vi "Main.vi"(11 "Module Admin":refnum<class "Delacor_lib_QMH_Cloneable Module Admin.lvclass">) -> ()   [LabVIEW 2020, in "reporting-device.lvlib"]
doc: "This template is based off of the Queued Message Handler design pattern and the Queued Message Handler project template that ships with LabVIEW.\n\nThe main difference is that the queue is private to this module and communication between modules is performed via Broadcast and Request events.\n\nRequest events are wrapped in public API methods and are handled in the Event Handling Loop (EHL) of this VI. Any module can register for Broadcast events sent by this module. The EHL generates messages based on user interface actions.\n\nThe Message Handling Loop (MHL) processes messages generated by the EHL, or by other messages. The messages are string values, so new messages can be added easily to the Message Cases case structure in the MHL. Each message cluster can also provide an optional value for Message Data, which is a variant that can be converted to whatever message-specific data is required.\n_____\nBased on DQMH Project Template 7.0.1.1316."
uses:
  reporting-device.lvlib
  <vilib>/Delacor/Delacor QMH/Libraries/Cloneable Module Admin_class/Delacor_lib_QMH_Cloneable Module Admin.lvclass
  C:/Program Files (x86)/National Instruments/LabVIEW 2020/vi.lib/Delacor/Delacor QMH/Libraries/Module Admin_class/Delacor_lib_QMH_Module Admin.lvclass
  <vilib>/Delacor/Delacor QMH/Libraries/Cloneable Module Admin_class/Delacor_lib_QMH_Cloneable Module Admin.lvclass/Delacor_lib_QMH_Cloneable Module Admin.ctl
  <vilib>/Wovalab/Utilities/Helper Loop Periodic Timing/Helper Loop Periodic Timing.lvclass/Helper Loop Periodic Timing.ctl
  <userlib>/Zaphiro/GTools/Redis/Sources/Redis/Redis.lvclass/Redis.ctl
  Stop Argument--cluster.ctl
  <vilib>/Delacor/Delacor QMH/Libraries/Message Queue_class/Delacor_lib_QMH_Message Queue.lvclass/Delacor_lib_QMH_Message Queue.ctl
  <vilib>/Delacor/Delacor QMH/Libraries/Module Admin_class/Delacor_lib_QMH_Module Admin.lvclass/Delacor_lib_QMH_Module Admin.ctl
  connect Argument--cluster.ctl
  connect (Reply Payload)--cluster.ctl
  start-publishing Argument--cluster.ctl
  start-publishing (Reply Payload)--cluster.ctl
  set-reporting-device Argument--cluster.ctl
  set-reporting-device (Reply Payload)--cluster.ctl
  <vilib>/Utility/miscctls.llb/LVPointTypeDef.ctl
  <vilib>/Delacor/Delacor QMH/Libraries/Cloneable Module Admin_class/Delacor_lib_QMH_Get Module ID.vi
  <vilib>/Delacor/Delacor QMH/Libraries/Message Queue_class/Delacor_lib_QMH_Enqueue Message (Single).vi
  <vilib>/Delacor/Delacor QMH/Libraries/Module Admin_class/Delacor_lib_QMH_Get External Launch.vi
  <userlib>/Zaphiro/GTools/Time/public/convert lv time to unix-scalar__ZGTools.vi
  <vilib>/Wovalab/Utilities/Helper Loop Periodic Timing/U32 Max Value--constant.vi
  <userlib>/Zaphiro/GTools/Redis/Sources/Redis/Hashes/HSET.vi
  <userlib>/Zaphiro/GTools/Redis/Sources/Redis/Keys/EXPIRE.vi
  <vilib>/Wovalab/Utilities/Helper Loop Periodic Timing/Update Last Execution Time.vi
  <vilib>/Wovalab/Utilities/Helper Loop Periodic Timing/Stop Helper Loop.vi
  <vilib>/Wovalab/Utilities/Helper Loop Periodic Timing/Stop Helper Loop Internal.vi
  <userlib>/Zaphiro/GTools/Redis/Sources/Redis/Connection/Send-command.vi
  <userlib>/Zaphiro/GTools/Redis/Sources/Redis/Connection/PING.vi
  <userlib>/Zaphiro/GTools/Redis/Sources/Redis/Connection/QUIT.vi
  <vilib>/Wovalab/Utilities/Helper Loop Periodic Timing/Loops Events AE.vi
  <vilib>/Wovalab/Utilities/Helper Loop Periodic Timing/Notify Monitoring Window.vi
  <vilib>/Wovalab/Utilities/Helper Loop Periodic Timing/Monitoring--global.vi
  <userlib>/Zaphiro/GTools/Redis/Sources/Redis/subVIs/LL_collect-response.vi
  <vilib>/Wovalab/Utilities/Helper Loop Periodic Timing/Helper Loop Periodic Timing.lvclass
  <userlib>/Zaphiro/GTools/Redis/Sources/Redis/Redis.lvclass
  <vilib>/Delacor/Delacor QMH/Libraries/Message Queue_class/Delacor_lib_QMH_Message Queue.lvclass
  <userlib>/Zaphiro/GTools/Time/time__ZGTools.lvlib
  <userlib>/Zaphiro/GTools/Time/public/convert unix time to lv-scalar__ZGTools.vi
panel:
  out "values":dbl[](array[numeric])
  out "timestamp":timestamp format="%^<%x %.3X>T utc"
  out "latest-ts":u64
  out "info":T1
  out "status":string
  out "connected":bool
  out "error out":errorcluster
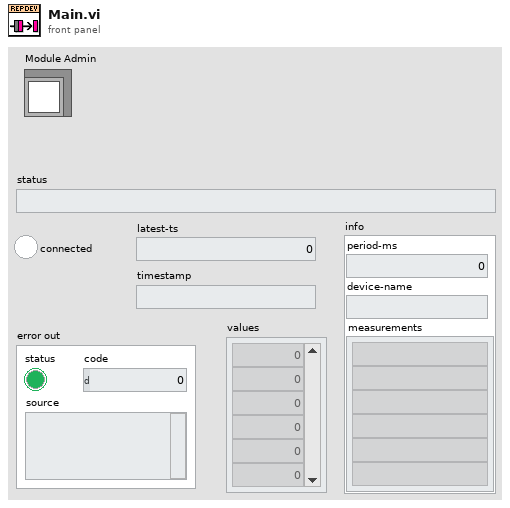
[diagram p1: front panel]
types:
  T1 = cluster{"period-ms":i32, "device-name":string, "measurements":string[]}
  T2 = typedef "reporting-device.lvlib/Request Events--cluster.ctl" = cluster{"Stop Module":refnum<user-event>, "Show Panel":refnum<user-event>, "Hide Panel":refnum<user-event>, "Show Diagram":refnum<user-event>, "Get Module Execution Status":refnum<user-event>, "connect":refnum<user-event>, "start-publishing":refnum<user-event>, "set-reporting-device":refnum<user-event>}
  T3 = typedef "reporting-device.lvlib/Module Data--cluster.ctl" = cluster{"clone-id":i32, "status":string, "dvr":cluster{"redis":refnum<data-value>}}
  T4 = enum32{"invalid lock state", "Not Locked", "Locked (No Password)", "Password-protected"}
  T5 = typedef "reporting-device.lvlib/Stop Argument--cluster.ctl" = cluster{"Module ID":i32, "Origin":string, "Exit via Stop Module Req?":bool, "Wait for Module to stop?":bool}
  T6 = typedef "reporting-device.lvlib/connect Argument--cluster.ctl" = cluster{"Module ID":i32, "flush":bool, "connection":cluster{"ip":string, "port":u16, "timeout":i32}, "Wait Notifier":refnum<notifier>, "wait for reply":bool}
  T7 = typedef "reporting-device.lvlib/start-publishing Argument--cluster.ctl" = cluster{"Module ID":i32, "Wait Notifier":refnum<notifier>, "wait for reply":bool}
  T8 = typedef "reporting-device.lvlib/set-reporting-device Argument--cluster.ctl" = cluster{"Module ID":i32, "measurement-list":string[], "period-ms":i32, "device-name":string, "Wait Notifier":refnum<notifier>, "wait for reply":bool}
  T9 = typedef "LVPointTypeDef.ctl" = cluster{"Horizontal":i16, "Vertical":i16}
  T10 = enum32{"Invalid", "Standard", "Closed", "Hidden", "Minimized", "Maximized"}
  T11 = typedef "reporting-device.lvlib/connect (Reply Payload)--cluster.ctl" = cluster{"Module ID":i32, "status":cluster{"reply-to-ping":bool, "pong":bool}, "error":errorcluster}
  T12 = typedef "reporting-device.lvlib/start-publishing (Reply Payload)--cluster.ctl" = cluster{"Module ID":i32, "ack":bool, "ts":u64, "error":errorcluster}
  T13 = typedef "reporting-device.lvlib/set-reporting-device (Reply Payload)--cluster.ctl" = cluster{"Module ID":i32, "ack":bool, "error":errorcluster}
  T14 = cluster{"output cluster":refnum<class "Redis.lvclass">}
  T15 = cluster{"period-ms":i32, "device-name":string, "measurement-list":string[]}
  T16 = cluster{u64, "device-name":string, "measurement-list":string[]}
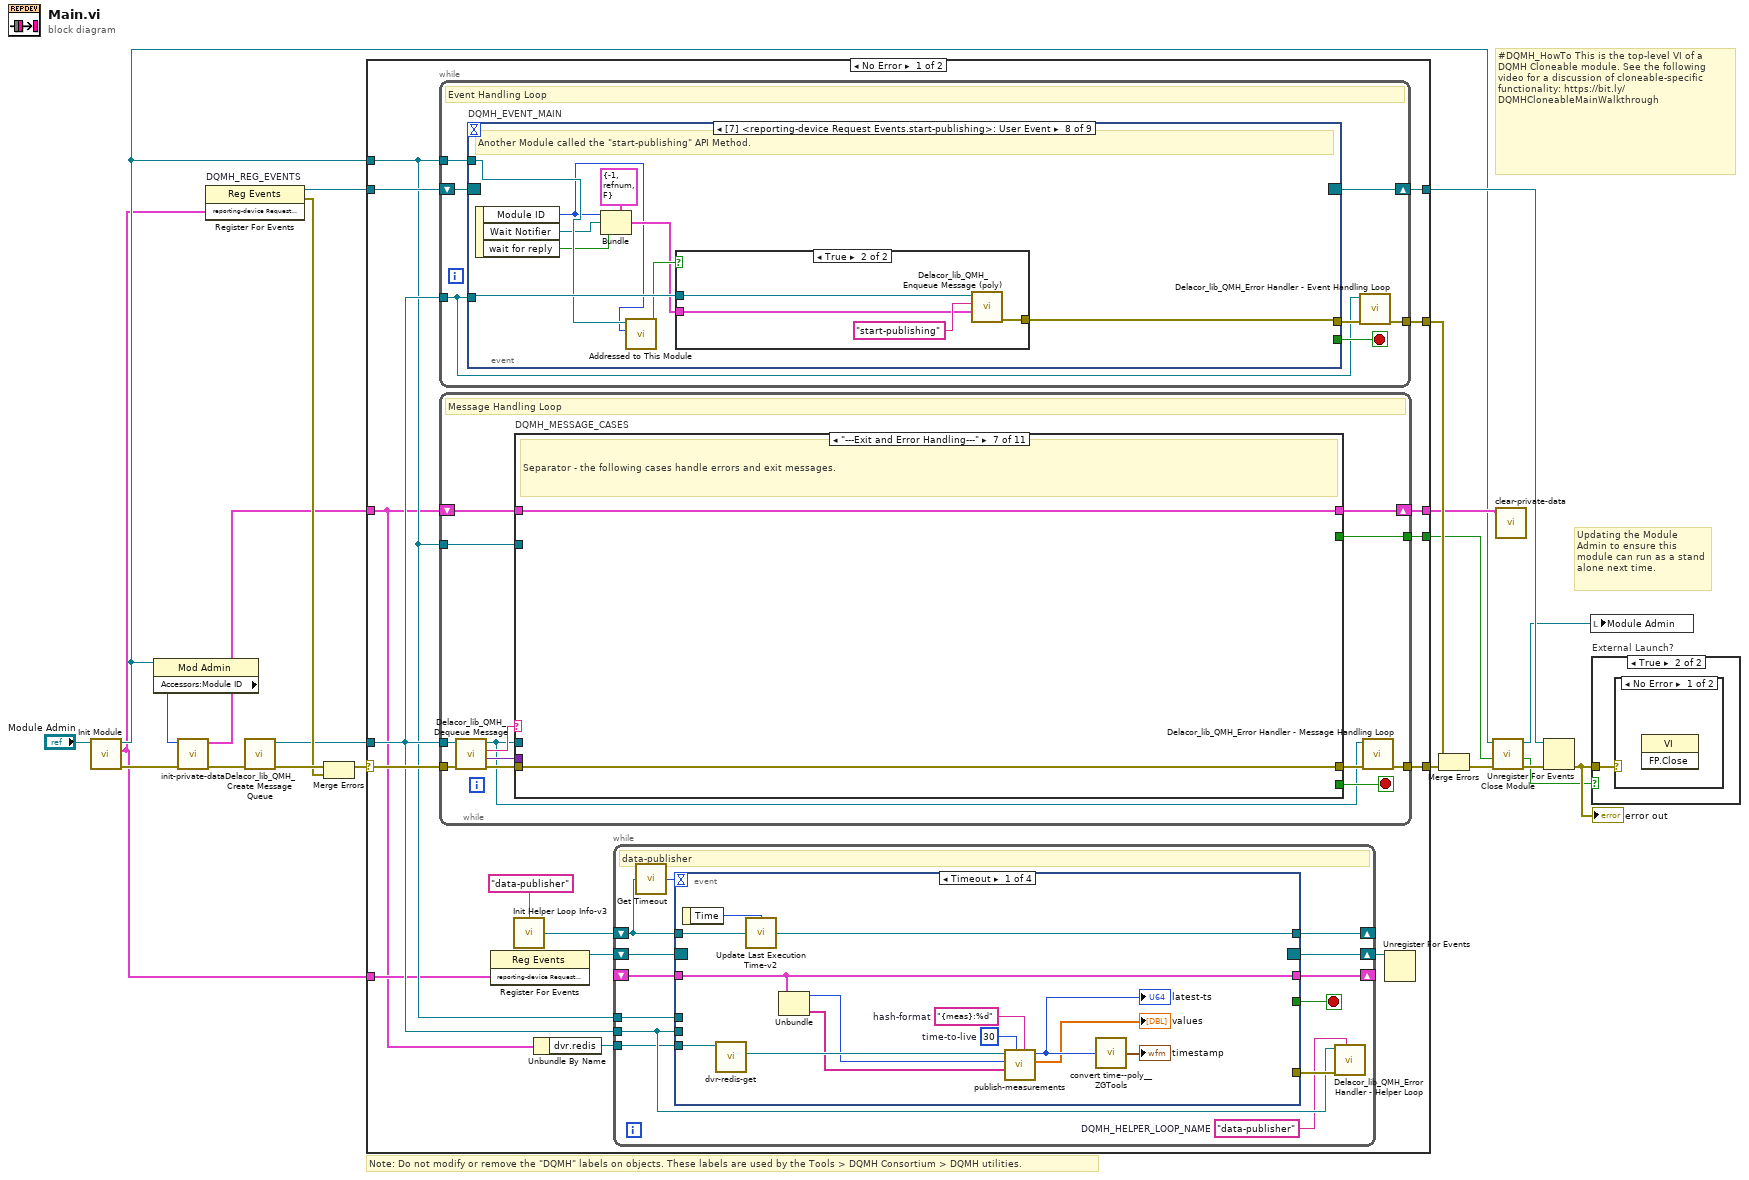
[diagram p0: block diagram]
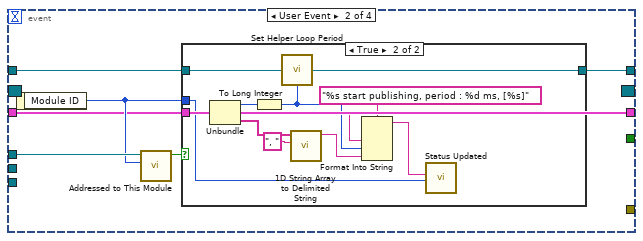
[diagram p2: hidden frame]
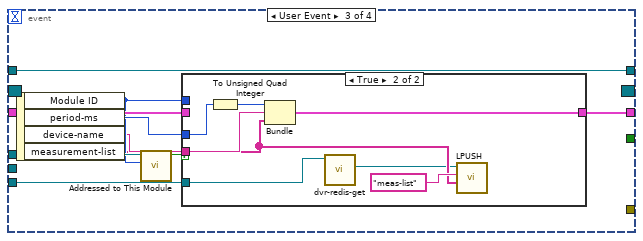
[diagram p4: hidden frame]
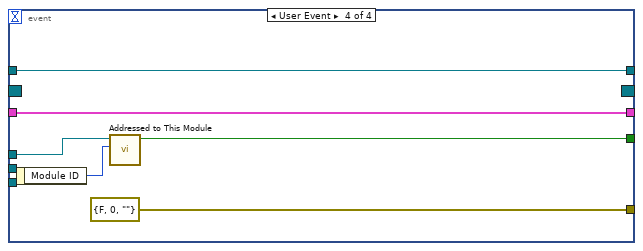
[diagram p6: hidden frame]
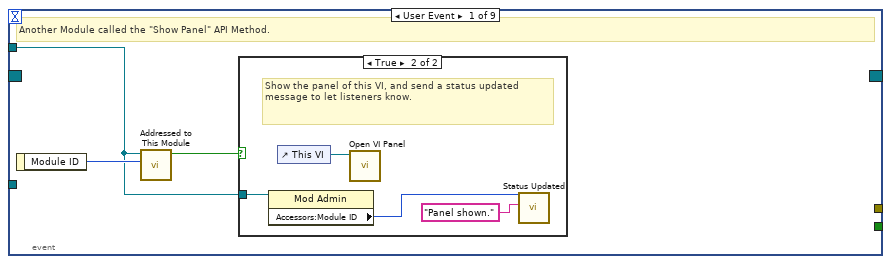
[diagram p7: hidden frame]
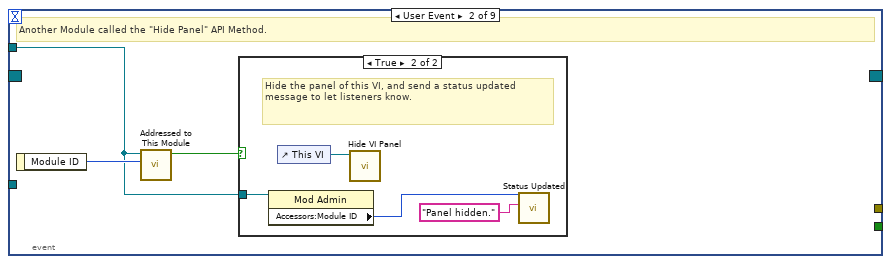
[diagram p9: hidden frame]
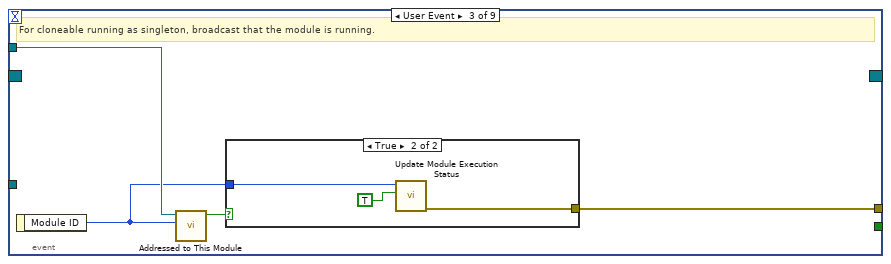
[diagram p11: hidden frame]
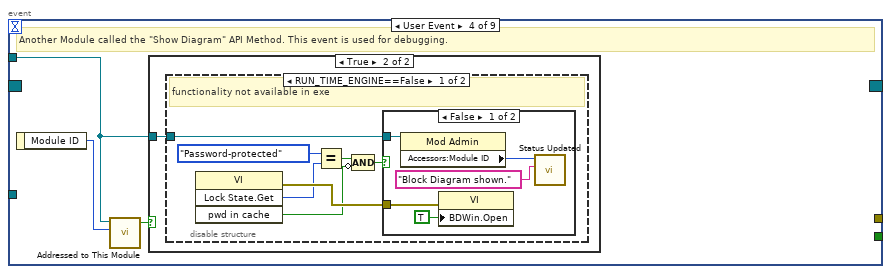
[diagram p13: hidden frame]
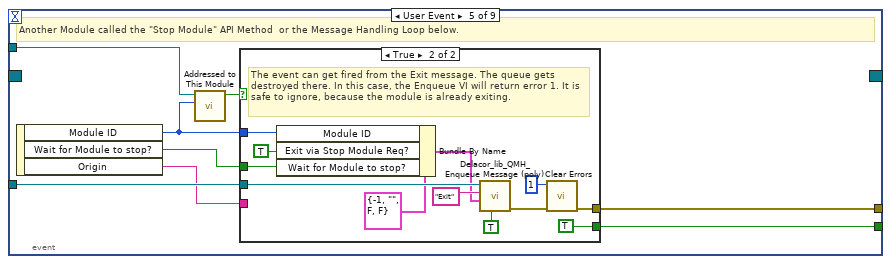
[diagram p17: hidden frame]
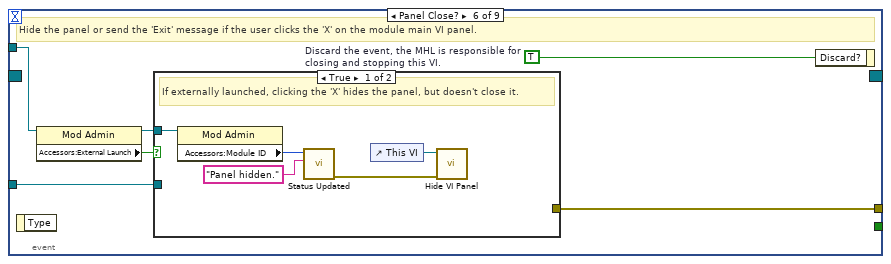
[diagram p19: hidden frame]
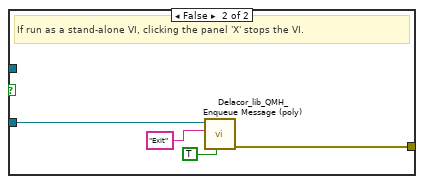
[diagram p20: hidden frame]
diagram:
  # "#DQMH_HowTo This is the top-level VI of a DQMH Cloneable module. See the following video for a discussion of cloneable-specific functionality: https://bit.ly/DQMHCloneableMainWalkthrough"
  # "Note: Do not modify or remove the \"DQMH\" labels on objects. These labels are used by the Tools > DQMH Consortium > DQMH utilities."
  # "Updating the Module Admin to ensure this module can run as a stand alone next time."
  n1 = call "Init Module.vi"("Cloneable Module Admin in"="Module Admin") -> ("error out"=w6:errorcluster, "reporting-device Request Events"=w1:T2, "Cloneable Module Admin out"=w3:refnum<class "Delacor_lib_QMH_Cloneable Module Admin.lvclass">)  [unwired: 8 in]
  n2 = property class="Mod Admin"(reference=w3) -> ("Accessors:Module ID"=w2:i32)  [unwired: 1 in, 2 out]
  n3 = call "init-private-data.vi"("error in (no error)"=w6, "clone-id"=w2) -> ("error out"=w5:errorcluster, "module-data"=w7:T3)  [unwired: 8 in]
  n4 = register-events "DQMH_REG_EVENTS"(w1) -> (reference out=w13:refnum<event-registration>, error out=w15:errorcluster)  [unwired: 2 in]
  n5 = call <vilib>:"Delacor_lib_QMH_Create Message Queue.vi"("error in"=w5) -> ("error out"=w17:errorcluster, "Message Queue"=w12:refnum<class "Delacor_lib_QMH_Message Queue.lvclass">)  [unwired: 9 in]
  n6 = Merge Errors(w17, w15) -> (w16:errorcluster)
  n7 = case shown="No Error" w16 {
    selector: w16 -> [w36 w409]
    tunnel: [w38 w408] -> w20
    tunnel: [w35 w407] -> w14
    tunnel: w13 -> [w34 w407]
    tunnel: w12 -> [w33 w400]
    tunnel: [w37 _] -> w21
    tunnel: w3 -> [w32 w403]
    tunnel: [w31 _] -> w9
    tunnel: w7 -> [w24 w399]
    tunnel: [w30 w399] -> w4
    tunnel: w1 -> [w29 _]
    frame No Error {
      n8 = while {
        tunnel: w33 -> [w109]
        shift-right: [w112] -> w35
        shift-left: w34 -> [w113]
        tunnel: [w114] -> w37
        tunnel: w32 -> [w110]
        stop <- w111 stop-if-true
        # "Event Handling Loop"
        n9 = event "DQMH_EVENT_MAIN" shown="[7] <reporting-device Request Events.start-publishing>: User Event" {
          selector: w113 -> [_ _ _ _ _ _ _ _ _]
          dyn-events: [_ _ _ _ _ _ _ _ _] -> w112
          timeout: _ -> [_ _ _ _ _ _ _ _ _]
          tunnel: [_ _ _ _ w156 _ _ _ _] -> w111
          tunnel: w109 -> [_ _ _ _ w159 w175 w198 w211 w227]
          tunnel: [_ _ w133 _ w160 w178 w188 w205 w216] -> w115
          tunnel: w110 -> [w116 w123 w131 w137 w158 w176 w196 w209 w225]
          event User Event {
            # "Another Module called the \"Show Panel\" API Method."
            n10 = event-data() -> ("Module ID"=w117:i32)  [unwired: 1 in]
            n11 = call "Addressed to This Module.vi"("Module ID from Argument"=w117, "Module Admin"=w116) -> ("Addressed to this instance?"=w118:bool)  [unwired: 8 in, 1 out]
            n12 = case shown="True" w118 {
              tunnel: w116 -> [_ w120]
              frame False {
              }
              frame True {
                # "Show the panel of this VI, and send a status updated message to let listeners know."
                n13 = property on="Property Node" class="Mod Admin"(reference=w120) -> ("Accessors:Module ID"=w119:i32)  [unwired: 1 in, 2 out]
                n14 = control-ref of="This VI"() -> (w122:refnum<vi>)
                n15 = call "Open VI Panel.vi"("VI"=w122) -> ()  [unwired: 10 in, 1 out]
                n16 = call "Status Updated.vi"("Status"="Panel shown." ("format string"), "Module ID"=w119) -> ()  [unwired: 9 in, 1 out]
              }
            }
          }
          event User Event {
            # "Another Module called the \"Hide Panel\" API Method."
            n17 = event-data() -> ("Module ID"=w124:i32)  [unwired: 1 in]
            n18 = call "Addressed to This Module.vi"("Module ID from Argument"=w124, "Module Admin"=w123) -> ("Addressed to this instance?"=w125:bool)  [unwired: 8 in, 1 out]
            n19 = case shown="True" w125 {
              tunnel: w123 -> [_ w127]
              frame False {
              }
              frame True {
                # "Hide the panel of this VI, and send a status updated message to let listeners know."
                n20 = property on="Property Node" class="Mod Admin"(reference=w127) -> ("Accessors:Module ID"=w126:i32)  [unwired: 1 in, 2 out]
                n21 = control-ref of="This VI"() -> (w129:refnum<vi>)
                n22 = call "Hide VI Panel.vi"("VI"=w129) -> ()  [unwired: 10 in, 1 out]
                n23 = call "Status Updated.vi"("Status"="Panel hidden." ("format string"), "Module ID"=w126) -> ()  [unwired: 9 in, 1 out]
              }
            }
          }
          event User Event {
            # "For cloneable running as singleton, broadcast that the module is running."
            n24 = event-data() -> ("Module ID"=w130:i32)  [unwired: 1 in]
            n25 = call "Addressed to This Module.vi"("Module ID from Argument"=w130, "Module Admin"=w131) -> ("Addressed to this instance?"=w132:bool)  [unwired: 8 in, 1 out]
            n26 = case shown="True" w132 {
              tunnel: [_ w136] -> w133
              tunnel: w130 -> [_ w135]
              frame False {
              }
              frame True {
                n27 = call "Update Module Execution Status.vi"("Running?"=TRUE, "Module ID"=w135) -> ("error out"=w136:errorcluster)  [unwired: 9 in]
              }
            }
          }
          event User Event {
            # "Another Module called the \"Show Diagram\" API Method. This event is used for debugging."
            n28 = event-data() -> ("Module ID"=w138:i32)  [unwired: 1 in]
            n29 = call "Addressed to This Module.vi"("Module ID from Argument"=w138, "Module Admin"=w137) -> ("Addressed to this instance?"=w139:bool)  [unwired: 8 in, 1 out]
            n30 = case shown="True" w139 {
              tunnel: w137 -> [_ w140]
              frame False {
              }
              frame True {
                n31 = disable-structure shown="RUN_TIME_ENGINE==False" {
                  disable-tunnel: w140 -> [w141 _]
                  frame condition #0 (active) {
                    # "functionality not available in exe"
                    n32 = invoke on="Invoke Node" class="VI" method="Lock State.Get"() -> (error out=w147:errorcluster, "Get Lock State"=w146:T4, "pwd in cache"=w143:bool)  [unwired: 4 in, 1 out]
                    n33 = Equal?(x=T4."Password-protected", y=w146) -> (x = y?=w144:bool)
                    n34 = Compound Arithmetic op=AND(w144, invert w143) -> (w142:bool)
                    n35 = case shown="False" w142 {
                      tunnel: w147 -> [w152 _]
                      tunnel: w141 -> [w149 _]
                      frame False {
                        n36 = property on="Property Node" class="Mod Admin"(reference=w149) -> ("Accessors:Module ID"=w148:i32)  [unwired: 1 in, 2 out]
                        n37 = property on="Property Node" class="VI"(error in=w152, "BDWin.Open"=TRUE ("Block Diagram Window:Open")) -> ()  [unwired: 1 in, 2 out]
                        n38 = call "Status Updated.vi"("Status"="Block Diagram shown." ("format string"), "Module ID"=w148) -> ()  [unwired: 9 in, 1 out]
                      }
                      frame True {
                        # "Password-protected VI, and the password is not in the cache. Do not show the diagram."
                      }
                    }
                  }
                  frame condition #1 {
                  }
                }
              }
            }
          }
          event User Event {
            # "Another Module called the \"Stop Module\" API Method  or the Message Handling Loop below."
            n39 = event-data() -> ("Module ID"=w154:i32, "Wait for Module to stop?"=w155:bool, "Origin"=w153:string)  [unwired: 1 in]
            n40 = call "Addressed to This Module.vi"("Module ID from Argument"=w154, "Module Admin"=w158) -> ("Addressed to this instance?"=w157:bool)  [unwired: 8 in, 1 out]
            n41 = case shown="True" w157 {
              tunnel: [_ w171] -> w160
              tunnel: w159 -> [_ w167]
              tunnel: [_ TRUE] -> w156
              tunnel: w155 -> [_ w162]
              tunnel: w154 -> [_ w164]
              tunnel: w153 -> [_ _]
              frame False {
              }
              frame True {
                # "The event can get fired from the Exit message. The queue gets destroyed there. In this case, the Enqueue VI will return error 1. It is safe to ignore, because the module is already exiting."
                n42 = Bundle By Name(cluster=T5 {"Module ID"=-1, "Origin"="", "Exit via Stop Module Req?"=FALSE, "Wait for Module to stop?"=FALSE} ("Stop Argument"), "Module ID"=w164, "Exit via Stop Module Req?"=TRUE, "Wait for Module to stop?"=w162) -> (w161:T5)
                n43 = call-poly <vilib>:"Delacor_lib_QMH_Enqueue Message (poly).vi"("Priority Message? (F)"=TRUE, "Message Data"=w161, "Message"="Exit", "Message Queue in"=w167) -> ("error out"=w172:errorcluster)  [unwired: 6 in, 1 out]
                n44 = call <vilib>:"Clear Errors.vi"("error in (no error)"=w172, "specific error code to clear (0: all)"=1) -> ("error out"=w171:errorcluster)  [unwired: 4 in, 1 out]
              }
            }
          }
          event Panel Close? {
            w177 = TRUE  # Discard the event, the MHL is responsible for closing and stopping this VI.
            # "Hide the panel or send the 'Exit' message if the user clicks the 'X' on the module main VI panel."
            n45 = event-data() -> ()  [unwired: 1 in, 1 out]
            n46 = property on="Property Node" class="Mod Admin"(reference=w176) -> (reference out=w173:refnum<class "Delacor_lib_QMH_Cloneable Module Admin.lvclass">, "Accessors:External Launch"=w174:bool)  [unwired: 1 in, 1 out]
            n47 = case shown="True" w174 {
              tunnel: w175 -> [_ w186]
              tunnel: [_ w187] -> w178
              tunnel: w173 -> [w181 _]
              frame True {
                # "If externally launched, clicking the 'X' hides the panel, but doesn't close it."
                n48 = property on="Property Node" class="Mod Admin"(reference=w181) -> ("Accessors:Module ID"=w180:i32)  [unwired: 1 in, 2 out]
                n49 = call "Status Updated.vi"("Status"="Panel hidden." ("format string"), "Module ID"=w180) -> ("error out"=w179:errorcluster)  [unwired: 9 in]
                n50 = control-ref of="This VI"() -> (w183:refnum<vi>)
                n51 = call "Hide VI Panel.vi"("error in"=w179, "VI"=w183) -> ()  [unwired: 9 in, 1 out]
              }
              frame False {
                # "If run as a stand-alone VI, clicking the panel 'X' stops the VI."
                n52 = call-poly <vilib>:"Delacor_lib_QMH_Enqueue Message (poly).vi"("Priority Message? (F)"=TRUE, "Message"="Exit", "Message Queue in"=w186) -> ("error out"=w187:errorcluster)  [unwired: 7 in, 1 out]
              }
            }
            n53 = event-data ("Event Filter Node")("Discard?"=w177) -> ()  [unwired: 1 in, 1 out]
          }
          event User Event {
            # "Another Module called the \"connect\" API Method."
            n54 = event-data() -> ("Module ID"=w193:i32, "flush"=w192:bool, "connection"=w191:cluster{"ip":string, "port":u16, "timeout":i32}, "Wait Notifier"=w190:refnum<notifier>, "wait for reply"=w189:bool)  [unwired: 1 in]
            n55 = Bundle(cluster=T6 {"Module ID"=-1, "flush"=FALSE, "connection"={"ip"="localhost", "port"=6379, "timeout"=1000}, "Wait Notifier"=refnum, "wait for reply"=FALSE} ("connect Argument"), "Module ID"=w193, "flush"=w192, "connection"=w191, "Wait Notifier"=w190, "wait for reply"=w189) -> (w194:T6)
            n56 = call "Addressed to This Module.vi"("Module ID from Argument"=w193, "Module Admin"=w196) -> ("Addressed to this instance?"=w197:bool)  [unwired: 8 in, 1 out]
            n57 = case shown="True" w197 {
              tunnel: w198 -> [_ w202]
              tunnel: w194 -> [_ w200]
              tunnel: [_ w199] -> w188
              frame False {
              }
              frame True {
                n58 = call-poly <vilib>:"Delacor_lib_QMH_Enqueue Message (poly).vi"("Message Data"=w200, "Message"="connect", "Message Queue in"=w202) -> ("error out"=w199:errorcluster)  [unwired: 7 in, 1 out]
              }
            }
          }
          event User Event {
            # "Another Module called the \"start-publishing\" API Method."
            n59 = event-data() -> ("Module ID"=w206:i32, "Wait Notifier"=w203:refnum<notifier>, "wait for reply"=w204:bool)  [unwired: 1 in]
            n60 = Bundle(cluster=T7 {"Module ID"=-1, "Wait Notifier"=refnum, "wait for reply"=FALSE} ("start-publishing Argument"), "Module ID"=w206, "Wait Notifier"=w203, "wait for reply"=w204) -> (w207:T7)
            n61 = call "Addressed to This Module.vi"("Module ID from Argument"=w206, "Module Admin"=w209) -> ("Addressed to this instance?"=w210:bool)  [unwired: 8 in, 1 out]
            n62 = case shown="True" w210 {
              tunnel: w211 -> [_ w215]
              tunnel: w207 -> [_ w213]
              tunnel: [_ w212] -> w205
              frame False {
              }
              frame True {
                n63 = call-poly <vilib>:"Delacor_lib_QMH_Enqueue Message (poly).vi"("Message Data"=w213, "Message"="start-publishing", "Message Queue in"=w215) -> ("error out"=w212:errorcluster)  [unwired: 7 in, 1 out]
              }
            }
          }
          event User Event {
            # "Another Module called the \"set-reporting-device\" API Method."
            n64 = event-data() -> ("Module ID"=w222:i32, "measurement-list"=w221:string[], "period-ms"=w220:i32, "device-name"=w219:string, "Wait Notifier"=w218:refnum<notifier>, "wait for reply"=w217:bool)  [unwired: 1 in]
            n65 = Bundle(cluster=T8 {"Module ID"=-1, "measurement-list"=[], "period-ms"=0, "device-name"="", "Wait Notifier"=refnum, "wait for reply"=FALSE} ("set-reporting-device Argument"), "Module ID"=w222, "measurement-list"=w221, "period-ms"=w220, "device-name"=w219, "Wait Notifier"=w218, "wait for reply"=w217) -> (w223:T8)
            n66 = call "Addressed to This Module.vi"("Module ID from Argument"=w222, "Module Admin"=w225) -> ("Addressed to this instance?"=w226:bool)  [unwired: 8 in, 1 out]
            n67 = case shown="True" w226 {
              tunnel: w227 -> [_ w231]
              tunnel: w223 -> [_ w229]
              tunnel: [_ w228] -> w216
              frame False {
              }
              frame True {
                n68 = call-poly <vilib>:"Delacor_lib_QMH_Enqueue Message (poly).vi"("Message Data"=w229, "Message"="set-reporting-device", "Message Queue in"=w231) -> ("error out"=w228:errorcluster)  [unwired: 7 in, 1 out]
              }
            }
          }
        }
        n69 = call-dynamic "Delacor_lib_QMH_Error Handler - Event Handling Loop.vi"("error in"=w115, "Message Queue in"=w109) -> ("dup error in"=w114:errorcluster)  [unwired: 8 in, 1 out]
      }
      n70 = while {
        tunnel: w33 -> [w232]
        shift-right: [w239] -> w30
        shift-left: w24 -> [w240]
        tunnel: w36 -> [w243]
        tunnel: [w241] -> w38
        tunnel: w32 -> [w234]
        tunnel: [w233] -> w31
        stop <- w238 stop-if-true
        # "Message Handling Loop"
        n71 = call-dynamic "Delacor_lib_QMH_Dequeue Message.vi"("error in"=w243, "Message Queue in"=w232) -> ("error out"=w242:errorcluster, "Message Data"=w236:variant, "Message"=w237:string, "Message Queue out"=w235:refnum<class "Delacor_lib_QMH_Message Queue.lvclass">)  [unwired: 6 in]
        n72 = case "DQMH_MESSAGE_CASES" shown="\"---Exit and Error Handling---\"" w237 {
          selector: w237 -> [_ _ _ _ _ _ _ _ _ _ w391]
          tunnel: w235 -> [_ _ _ _ _ _ _ w342 _ w379 _]
          tunnel: w242 -> [w263 w267 w292 w313 w331 w336 w338 w350 w366 w385 w397]
          tunnel: [w261 w267 w279 w305 w318 w335 w338 w346 w365 w380 w398] -> w244
          tunnel: w240 -> [w246 w266 w278 w300 w317 w334 w337 w340 w358 w370 w389]
          tunnel: [w254 w266 w278 w300 w317 w334 w337 w340 w358 w370 w389] -> w239
          tunnel: [_ _ _ _ _ _ _ _ _ w378 _] -> w238
          tunnel: w236 -> [_ _ w291 w312 w330 _ _ w345 _ w376 _]
          tunnel: w234 -> [w250 _ _ _ _ _ _ w344 _ w371 _]
          tunnel: [_ _ _ _ _ _ _ _ _ w374 _] -> w233
          frame "Initialize" {
            # "#CodeNeeded - Initialize the appearance of the front panel."
            # "#CodeNeeded - Initialize your state data here."
            # "Initialize - Any operation that needs to be done before the module can receive messages. Synchronize Caller Events.vi will inform Start Module.vi that the module has launched and is ready to receive messages. Module Did Init.vi will broadcast that the module initialized."
            n73 = call "Synchronize Caller Events.vi"("error in"=w263, "Module Admin"=w250) -> ("error out"=w262:errorcluster, "Module Admin out"=w249:refnum<class "Delacor_lib_QMH_Cloneable Module Admin.lvclass">)  [unwired: 8 in]
            n74 = property on="Property Node" class="Mod Admin"(reference=w249) -> ("Accessors:External Launch"=w251:bool)  [unwired: 1 in, 2 out]
            n75 = Unbundle By Name(w246) -> ("clone-id"=w245:i32)
            n76 = call "Module Name--constant.vi"("Module ID"=w245) -> ("Module Name"=w258:string)  [unwired: 10 in]
            n77 = property on="Property Node" class="VI"("Front Panel.Title"=w258) -> (reference out=w260:refnum<vi>, error out=w265:errorcluster)  [unwired: 2 in]
            n78 = Select(t=T10."Hidden" ("State"), s=w251, f=T10."Standard" ("State")) -> (s? t:f=w255:T10)
            n79 = invoke on="Invoke Node" class="VI" method="FP.Open"(reference=w260, error in=w265, "State"=w255) -> (reference out=w259:refnum<vi>, error out=w264:errorcluster)  [unwired: 2 in, 3 out]
            n80 = call "Module Name--constant.vi"("Module ID"=w245) -> ("Module Name"=w252:string)  [unwired: 10 in]
            n81 = Bundle By Name(cluster=w246, "status"="Initial Message" ("Initial Message")) -> (w254:T3)
            n82 = invoke on="Invoke Node" class="VI" method="FP.Center"(reference=w259, error in=w264) -> ()  [unwired: 1 in, 3 out]
            n83 = property on="Pane" class="Pane"("Origin"=T9 {"Horizontal"=0, "Vertical"=0}) -> ()  [unwired: 2 in, 2 out]
            n84 = call "Module Did Init.vi"("error in"=w262, "Initialized?"=TRUE, "Origin"=w252, "Module ID"=w245) -> ("error out"=w261:errorcluster)  [unwired: 7 in]
          }
          frame "---Module Specific---" {
            # "Separator -- The following cases handle messages specific to this Module."
          }
          frame "connect" {
            w280 = TRUE  # #oneday
            # "connect to a redis instance"
            n85 = Variant To Data(error in=w292, type=T6 {"Module ID"=-1, "flush"=FALSE, "connection"={"ip"="localhost", "port"=6379, "timeout"=1000}, "Wait Notifier"=refnum, "wait for reply"=FALSE} ("connect Argument"), Variant=w291) -> (data=w289:T6, error out=w279:errorcluster)
            n86 = Unbundle By Name(w289) -> ("flush"=w284:bool, "connection"=w283:cluster{"ip":string, "port":u16, "timeout":i32}, "Wait Notifier"=w288:refnum<notifier>, "wait for reply"=w287:bool)
            n87 = Unbundle By Name(w283) -> ("ip"=w274:string, "port"=w273:u16, "timeout"=w282:i32)
            n88 = Unbundle By Name(w278) -> ("clone-id"=w275:i32, "dvr.redis"=w277:refnum<data-value>)
            n89 = call <userlib>:"Open_Redis.vi"("Flush Stack befor each cmd"=w284, "Tcp timeout ms"=w282, "Port"=w273, "Host"=w274) -> ("error out"=w281:errorcluster, "connection-ok"=w272:bool, "output cluster"=w276:refnum<class "Redis.lvclass">)  [unwired: 5 in]
            "connected" <- w272
            n90 = case shown="True" w272 {
              tunnel: w277 -> [_ w293]
              tunnel: w276 -> [_ w294]
              frame False {
              }
              frame True {
                n91 = in-place {
                  in-place-border: w294 -> [w296]
                  n92 = in-place-dvr #1(w293) -> ()  [unwired: 2 out]
                  n93 = Bundle("output cluster"=w296) -> (w295:T14)  [unwired: 1 in]
                  n94 = in-place-dvr #1(w295) -> ()  [unwired: 2 out]
                }
              }
            }
            n95 = Select(t="connected to %s:%d" ("format string"), s=w272, f="failed to connect to %s:%d" ("format string")) -> (s? t:f=w269:string)
            n96 = Format Into String(format string=w269, w274, w273) -> (resulting string=w268:string)  [unwired: 2 in, 1 out]
            "status" <- w268
            n97 = Bundle By Name(cluster=T11 {"Module ID"=-1, "status"={"reply-to-ping"=FALSE, "pong"=FALSE}, "error"={"status"=FALSE, "code"=0, "source"=""}} ("connect (Reply Payload)"), "Module ID"=w275, "status.reply-to-ping"=w280, "status.pong"=w272, "error"=w281) -> (w286:T11)
            n98 = call "Status Updated.vi"("Status"=w268, "Module ID"=w275) -> ()  [unwired: 9 in, 1 out]
            n99 = case "DQMH_FIRE_NOTIFIER" shown="True" w287 {
              tunnel: w288 -> [_ w298]
              tunnel: w286 -> [_ w297]
              frame False {
              }
              frame True {
                n100 = Send Notification(notification=w297, notifier=w298) -> ()  [unwired: 1 in, 2 out]
              }
            }
          }
          frame "start-publishing" {
            # "start data publishing at given period the given meausrement list"
            n101 = Variant To Data(error in=w313, type=T7 {"Module ID"=-1, "Wait Notifier"=refnum, "wait for reply"=FALSE} ("start-publishing Argument"), Variant=w312) -> (data=w310:T7, error out=w305:errorcluster)
            n102 = Unbundle By Name(w310) -> ("Wait Notifier"=w309:refnum<notifier>, "wait for reply"=w308:bool)
            n103 = Unbundle By Name(w300) -> ("clone-id"=w299:i32)
            n104 = Get Date/Time In Seconds() -> (seconds since 1Jan1904=w302:timestamp)
            n105 = call-poly <userlib>:"convert time--poly__ZGTools.vi"("labview-timestamp"=w302) -> ("unix-time"=w301:u64)  [unwired: 8 in]
            n106 = Bundle By Name(cluster=T12 {"Module ID"=-1, "ack"=FALSE, "ts"=0, "error"={"status"=FALSE, "code"=0, "source"=""}} ("start-publishing (Reply Payload)"), "Module ID"=w299, "ack"=TRUE, "ts"=w301, "error"=errorcluster {"status"=FALSE, "code"=0, "source"=""}) -> (w307:T12)
            n107 = case "DQMH_FIRE_NOTIFIER" shown="True" w308 {
              tunnel: w309 -> [_ w315]
              tunnel: w307 -> [_ w314]
              frame False {
              }
              frame True {
                n108 = Send Notification(notification=w314, notifier=w315) -> ()  [unwired: 1 in, 2 out]
              }
            }
          }
          frame "set-reporting-device" {
            n109 = Variant To Data(error in=w331, type=T8 {"Module ID"=-1, "measurement-list"=[], "period-ms"=0, "device-name"="", "Wait Notifier"=refnum, "wait for reply"=FALSE} ("set-reporting-device Argument"), Variant=w330) -> (data=w328:T8, error out=w318:errorcluster)
            n110 = Unbundle By Name(w328) -> ("measurement-list"=w320:string[], "period-ms"=w322:i32, "device-name"=w321:string, "Wait Notifier"=w327:refnum<notifier>, "wait for reply"=w326:bool)
            n111 = Unbundle By Name(w317) -> ("clone-id"=w316:i32)
            n112 = Bundle("period-ms"=w322, "device-name"=w321, "measurement-list"=w320) -> (→"info":T15)  [unwired: 1 in]
            n113 = Bundle By Name(cluster=T13 {"Module ID"=-1, "ack"=FALSE, "error"={"status"=FALSE, "code"=0, "source"=""}} ("set-reporting-device (Reply Payload)"), "Module ID"=w316, "ack"=TRUE) -> (w325:T13)
            n114 = case "DQMH_FIRE_NOTIFIER" shown="True" w326 {
              tunnel: w327 -> [_ w333]
              tunnel: w325 -> [_ w332]
              frame False {
              }
              frame True {
                n115 = Send Notification(notification=w332, notifier=w333) -> ()  [unwired: 1 in, 2 out]
              }
            }
          }
          frame "---Copy This Frame---" {
            # "Duplicate this frame when creating new messages.  Change this comment in the duplicated frame to describe this message."
            n116 = Merge Errors(w336) -> (w335:errorcluster)
          }
          frame "---Exit and Error Handling---" {
            # "Separator - the following cases handle errors and exit messages."
          }
          frame "Error" {
            # "#CodeRecommended - If the module is running in standalone mode (External Launch = FALSE), this code will pop up an error dialog and call the 'Exit' message if an error occurs. Add more fine-grained error management here."
            # "Error - Check the error message data and respond accordingly. This message is sent by the \"Error Handler\" VIs at the end of each loop in this application."
            n117 = property on="Property Node" class="Mod Admin"(reference=w344) -> ("Accessors:External Launch"=w343:bool)  [unwired: 1 in, 2 out]
            n118 = Variant To Data(error in=w350, type=errorcluster {"status"=FALSE, "code"=0, "source"=""} ("error constant"), Variant=w345) -> (data=w341:errorcluster, error out=w348:errorcluster)
            n119 = Unbundle By Name(w340) -> ("clone-id"=w339:i32)
            n120 = local write "error out"(w341) -> ()
            n121 = call "Error Reported.vi"("Error"=w341, "Module ID"=w339) -> ()  [unwired: 9 in, 1 out]
            n122 = case shown="False" w343 {
              tunnel: [w355 _] -> w347
              tunnel: w342 -> [w353 _]
              tunnel: w341 -> [w354 _]
              frame False {
                n123 = disable-structure shown="Default" {
                  disable-tunnel: w354 -> [w356 _]
                  frame condition #0 (active) {
                    # "If the module is running standalone, then pop up an error dialog and call the \"Exit\" message."
                    n124 = call <vilib>:"Simple Error Handler.vi"("error in (no error)"=w356) -> ()  [unwired: 4 in, 5 out]
                  }
                  frame condition #1 {
                    # "To prevent the Simple Error Handler VI from being loaded (e.g. when deploying to a Real-Time target), add the Conditional Disable Symbol \"DQMH_Disable_SEH\" to your project and set it to TRUE."
                  }
                }
                n125 = call-poly <vilib>:"Delacor_lib_QMH_Enqueue Message (poly).vi"("Priority Message? (F)"=TRUE, "Message"="Exit", "Message Queue in"=w353) -> ("error out"=w355:errorcluster)  [unwired: 7 in, 1 out]
              }
              frame True {
                # "If the module was launched externally, calling the Error Reported broadcast VI is the only action performed by the \"Error\" message. The module's caller can then process the error appropriately."
              }
            }
            n126 = Merge Errors(w348, w347) -> (w346:errorcluster)
          }
          frame "Simulate MHL Error" {
            # "#DQMH_HowTo The 'Simulate MHL Error' button  illustrates how the MHL handles errors. This event is instructional in nature and can be removed."
            # "Simulate an error occurring at the MHL"
            n127 = Unbundle By Name(w358) -> ("clone-id"=w357:i32)
            n128 = call "Module Name--constant.vi"("Module ID"=w357) -> ("Module Name"=w360:string)  [unwired: 10 in]
            n129 = Format Into String(format string="Simulated error originating at Message Handling Loop in %s", w360) -> (resulting string=w361:string)  [unwired: 2 in, 1 out]
            n130 = call <vilib>:"Error Cluster From Error Code.vi"("show call chain? (False)"=TRUE, "error message (\"\")"=w361, "error code (0)"=5001) -> ("error out"=w364:errorcluster)  [unwired: 6 in]
            n131 = Merge Errors(w366, w364) -> (w365:errorcluster)
          }
          frame "Exit" {
            w377 = 91  # 91: not all Exit messages will have an argument
            w378 = TRUE  # Stop the VI
            # "Release the message queue reference"
            # "#CodeNeeded - Add any required cleanup code here."
            # "Exit - Exit the application."
            n132 = Variant To Data(error in=w385, type=T5 {"Module ID"=-1, "Origin"="", "Exit via Stop Module Req?"=FALSE, "Wait for Module to stop?"=FALSE} ("Stop Argument"), Variant=w376) -> (data=w373:T5, error out=w381:errorcluster)
            n133 = call <vilib>:"Clear Errors.vi"("error in (no error)"=w381, "specific error code to clear (0: all)"=w377) -> ("error out"=w384:errorcluster)  [unwired: 4 in, 1 out]
            n134 = Unbundle By Name(w370) -> ("clone-id"=w369:i32, "dvr.redis"=w368:refnum<data-value>)
            n135 = control-ref of="This VI"() -> (w372:refnum<vi>)
            n136 = call-dynamic "Delacor_lib_QMH_Release Message Queue.vi"("error in"=w384, "Message Queue"=w379) -> ("error out"=w383:errorcluster)  [unwired: 9 in]
            n137 = call "Handle Exit.vi"("Stop Argument"=w373, "Module Admin in"=w371, "VI reference"=w372) -> ("error out"=w382:errorcluster, "Wait for Stop?"=w374:bool)  [unwired: 7 in]
            n138 = in-place {
              in-place-border: [w386] -> w367
              n139 = in-place-dvr #2(w368) -> (w387:T14)  [unwired: 1 out]
              n140 = Unbundle(w387) -> ("output cluster"=w386:refnum<class "Redis.lvclass">)
              n141 = in-place-dvr #2() -> ()  [unwired: 1 in, 2 out]
            }
            n142 = Merge Errors(w383, w382) -> (w380:errorcluster)
            n143 = call "Error Reported.vi"("Error"=w380, "Module ID"=w369) -> ()  [unwired: 9 in, 1 out]
            n144 = call <userlib>:"Close_Redis.vi"("Redis.lvclass in"=w367) -> ()  [unwired: 9 in, 2 out]
          }
          frame Default {
            # "'Default' case only runs if there is a message that isn't defined in any of the other cases.  Output a programming error."
            n145 = Unbundle By Name(w389) -> ("clone-id"=w388:i32)
            n146 = call "Module Name--constant.vi"("Module ID"=w388) -> ("Module Name"=w390:string)  [unwired: 10 in]
            n147 = Format Into String(format string="The invalid message string \"%s\" was received in the Message Handling Loop for module \"%s\".", w391, w390) -> (resulting string=w393:string)  [unwired: 2 in, 1 out]
            n148 = call <vilib>:"Error Cluster From Error Code.vi"("show call chain? (False)"=TRUE, "error message (\"\")"=w393, "error code (0)"=1) -> ("error out"=w396:errorcluster)  [unwired: 6 in]
            n149 = Merge Errors(w397, w396) -> (w398:errorcluster)
          }
        }
        n150 = call-dynamic "Delacor_lib_QMH_Error Handler - Message Handling Loop.vi"("error in"=w244, "Message Queue in"=w235) -> ("dup error in"=w241:errorcluster)  [unwired: 8 in, 1 out]
      }
      n151 = register-events ("DQMH_HELPER_REGFOREVENTS")(w29) -> (reference out=w27:refnum<event-registration>)  [unwired: 2 in, 1 out]
      n152 = call <vilib>:"Init Helper Loop Info-v3.vi"("Loop Name (\"\": Caller VI)"="data-publisher" ("Loop Name (\"\": Caller VI)")) -> ("Helper Loop Periodic Timing"=w25:refnum<class "Helper Loop Periodic Timing.lvclass">)  [unwired: 1 in]
      n153 = Unbundle By Name(w24) -> ("dvr.redis"=w23:refnum<data-value>)
      n154 = while "DQMH_HELPER_LOOP" {
        shift-right: [w51] -> _
        shift-left: w25 -> [w43]
        shift-right: [w49] -> w28
        shift-left: w27 -> [w50]
        tunnel: w33 -> [w46]
        tunnel: w32 -> [w44]
        shift-right: [w41] -> _
        shift-left: _ -> [w40]
        tunnel: w23 -> [w39]
        stop <- w48 stop-if-true
        w45 = "data-publisher"  # DQMH_HELPER_LOOP_NAME
        # "data-publisher"
        n155 = call <vilib>:"Get Timeout.vi"("Helper Loop Periodic Timing"=w43) -> ("Timeout (ms)"=w42:i32)  [unwired: 12 in, 2 out]
        n156 = event "DQMH_HELPER_EVENT_STRUCTURE" shown="[0] Timeout" {
          selector: w50 -> [_ _ _ _]
          dyn-events: [_ _ _ _] -> w49
          timeout: w42 -> [_ _ _ _]
          tunnel: w43 -> [w63 w70 w87 w108]
          tunnel: [w64 w69 w87 w108] -> w51
          tunnel: [_ _ _ w105] -> w48
          tunnel: [_ _ _ errorcluster {"status"=FALSE, "code"=0, "source"=""} ("error constant")] -> w47
          tunnel: w46 -> [_ _ _ _]
          tunnel: w44 -> [_ w68 w93 w106]
          tunnel: [w62 w65 w90 w103] -> w41
          tunnel: w39 -> [w61 _ w84 _]
          tunnel: w40 -> [w62 w65 w89 w103]
          event Timeout {
            w57 = "{meas}:%d"  # hash-format
            w58 = u64 30  # time-to-live
            n157 = event-data() -> ("Time"=w54:u32)  [unwired: 1 in]
            n158 = call "dvr-redis-get.vi"("redis-dvr"=w61) -> ("Redis out"=w60:refnum<class "Redis.lvclass">)  [unwired: 10 in]
            n159 = call <vilib>:"Update Last Execution Time-v2.vi"("Time"=w54, "Helper Loop Periodic Timing in"=w63) -> ("Helper Loop Periodic Timing out"=w64:refnum<class "Helper Loop Periodic Timing.lvclass">)  [unwired: 12 in, 1 out]
            n160 = Unbundle(w62) -> (w55:u64, "measurement-list"=w59:string[])  [unwired: 1 out]
            n161 = call "publish-measurements.vi"("hash-format"=w57, "ttl"=w58, "measurement-list"=w59, "period"=w55, "Redis in"=w60) -> ("values"=→"values":dbl[], "unix-time"=w53:u64)  [unwired: 4 in, 1 out]
            "latest-ts" <- w53
            n162 = call-poly <userlib>:"convert time--poly__ZGTools.vi"("unix-time"=w53) -> ("labview-timestamp"=→"timestamp":timestamp)  [unwired: 8 in]
          }
          event User Event {
            n163 = event-data() -> ("Module ID"=w66:i32)  [unwired: 1 in]
            n164 = call "Addressed to This Module.vi"("Module ID from Argument"=w66, "Module Admin"=w68) -> ("Addressed to this instance?"=w67:bool)  [unwired: 8 in, 1 out]
            n165 = case shown="True" w67 {
              tunnel: w70 -> [w71 w83]
              tunnel: [w71 w82] -> w69
              tunnel: w65 -> [_ w76]
              tunnel: w66 -> [_ w77]
              frame False {
              }
              frame True {
                n166 = Unbundle(w76) -> (w75:u64, "device-name"=w74:string, "measurement-list"=w73:string[])
                n167 = To Long Integer(number=w75) -> (32bit integer=w72:i32)
                n168 = call <vilib>:"Set Helper Loop Period.vi"("Period (ms)"=w72, "Helper Loop Periodic Timing in"=w83) -> ("Helper Loop Periodic Timing out"=w82:refnum<class "Helper Loop Periodic Timing.lvclass">)  [unwired: 13 in]
                n169 = call <vilib>:"1D String Array to Delimited String.vi"("delimiter"=", ", "string array"=w73) -> ("delimited string"=w80:string)  [unwired: 9 in]
                n170 = Format Into String(format string="%s start publishing, period : %d ms, [%s]", w74, w72, w80) -> (resulting string=w81:string)  [unwired: 2 in, 1 out]
                n171 = call "Status Updated.vi"("Status"=w81, "Module ID"=w77) -> ()  [unwired: 9 in, 1 out]
              }
            }
          }
          event User Event {
            n172 = event-data() -> ("Module ID"=w88:i32, "period-ms"=w91:i32, "device-name"=w86:string, "measurement-list"=w85:string[])  [unwired: 1 in]
            n173 = call "Addressed to This Module.vi"("Module ID from Argument"=w88, "Module Admin"=w93) -> ("Addressed to this instance?"=w92:bool)  [unwired: 8 in, 1 out]
            n174 = case shown="True" w92 {
              tunnel: w91 -> [_ w101]
              tunnel: [w94 w102] -> w90
              tunnel: w89 -> [w94 _]
              tunnel: w88 -> [_ _]
              tunnel: w86 -> [_ w100]
              tunnel: w85 -> [_ w96]
              tunnel: w84 -> [_ w98]
              frame False {
              }
              frame True {
                n175 = To Unsigned Quad Integer(1:w101) -> (0:w99:u64)
                n176 = Bundle(w99, "device-name"=w100, "measurement-list"=w96) -> (w102:T16)  [unwired: 1 in]
                n177 = call "dvr-redis-get.vi"("redis-dvr"=w98) -> ("Redis out"=w95:refnum<class "Redis.lvclass">)  [unwired: 10 in]
                n178 = call <userlib>:"LPUSH.vi"("Elements"=w96, "Key"="meas-list", "Redis.lvclass in"=w95) -> ()  [unwired: 6 in, 3 out]
              }
            }
          }
          event User Event {
            n179 = event-data() -> ("Module ID"=w104:i32)  [unwired: 1 in]
            n180 = call "Addressed to This Module.vi"("Module ID from Argument"=w104, "Module Admin"=w106) -> ("Addressed to this instance?"=w105:bool)  [unwired: 8 in, 1 out]
          }
        }
        n181 = call-dynamic "Delacor_lib_QMH_Error Handler - Helper Loop.vi"("Error Debug"=w45, "error in"=w47, "Message Queue in"=w46) -> ()  [unwired: 7 in, 2 out]
      }
      n182 = Unregister For Events(event registration refnum=w28) -> ()  [unwired: 1 in, 1 out]
    }
    frame Error {
      n183 = call "Synchronize Caller Events.vi"("Module Admin"=w403) -> ("Module Admin out"=w402:refnum<class "Delacor_lib_QMH_Cloneable Module Admin.lvclass">)  [unwired: 9 in, 1 out]
      n184 = property on="Property Node" class="Mod Admin"(reference=w402) -> ("Accessors:Module ID"=w401:i32)  [unwired: 1 in, 2 out]
      n185 = call-dynamic "Delacor_lib_QMH_Release Message Queue.vi"("error in"=w409, "Message Queue"=w400) -> ("error out"=w408:errorcluster)  [unwired: 9 in]
      n186 = call "Module Name--constant.vi"("Module ID"=w401) -> ("Module Name"=w406:string)  [unwired: 10 in]
      n187 = Format Into String(format string="An error occurred during initialization. %s is no longer running.", w406) -> (resulting string=w404:string)  [unwired: 2 in, 1 out]
      n188 = call "Error Reported.vi"("Additional Information"=w404, "Error"=w408, "Module ID"=w401) -> ()  [unwired: 8 in, 1 out]
    }
  }
  n189 = Merge Errors(w21, w20) -> (w22:errorcluster)
  n190 = call "Close Module.vi"("error in"=w22, "Wait for stop?"=w9, "Module Admin in"=w3) -> ("error out"=w19:errorcluster, "External Launch"=w8:bool, "Module Admin out"=w10:refnum<class "Delacor_lib_QMH_Cloneable Module Admin.lvclass">)  [unwired: 6 in]
  n191 = call "clear-private-data.vi"("module-data"=w4) -> ()  [unwired: 10 in, 1 out]
  n192 = Unregister For Events(event registration refnum=w14, error in=w19) -> (error out=w18:errorcluster)
  "error out" <- w18
  n193 = local write "Module Admin"(w10) -> ()
  n194 = case "External Launch?" shown="True" w8 {
    tunnel: w18 -> [_ w410]
    frame False {
    }
    frame True {
      n195 = case shown="No Error" w410 {
        frame No Error {
          n196 = invoke class="VI" method="FP.Close"() -> ()  [unwired: 3 in, 3 out]
        }
        frame Error {
          n197 = invoke class="VI" method="FP.Open"("Activate"=TRUE ("Activate?")) -> ()  [unwired: 4 in, 5 out]
        }
      }
    }
  }
